vi "Pusher_Client_GetConnectionID.vi"(8 "error in (no error)":errorcluster, 11 "Client in":refnum<class "Client.lvclass">) -> (0 "error out":errorcluster, 3 "connectionID":refnum<k5>)   [LabVIEW 2009, in "Client.lvclass"]
uses:
  Client.lvclass
  Client.lvclass/Client.ctl
panel:
  out "Client out":refnum<class "Client.lvclass">
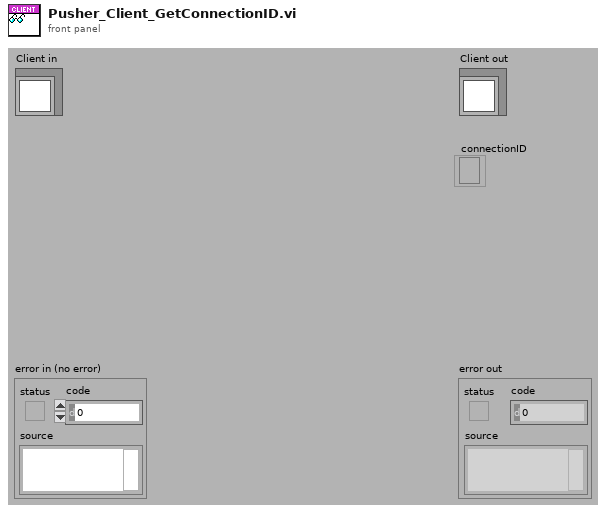
[diagram p1: front panel]
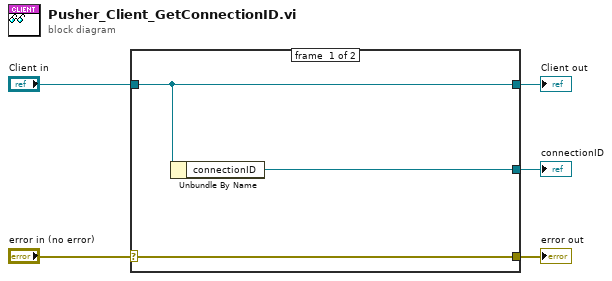
[diagram p0: block diagram]
diagram:
  n1 = case shown="No Error" "error in (no error)" {
    selector: "error in (no error)" -> [w8 w9]
    tunnel: [w8 w9] -> w4
    tunnel: [w7 w10] -> w2
    tunnel: "Client in" -> [w7 w10]
    tunnel: [w6 _] -> w1
    frame #0 {
      n2 = Unbundle By Name(w7) -> ("connectionID"=w6:refnum<k5>)
    }
    frame #1 {
    }
  }
  "error out" <- w4
  "Client out" <- w2
  "connectionID" <- w1
